vi "TBM.GetCallerCoordinates.vi"(8 "error in (no error)":errorcluster, 11 "Control in":refnum<vi>) -> (0 "error out":errorcluster, 1 "FP Screen Bounds":T1, 2 "Pane Color":u32, 3 "Ctrl Screen Bounds":T1)   [LabVIEW 2013, in "ToolbarMenu.lvlib"]
uses:
  ToolbarMenu.lvlib
  <vilib>/Utility/miscctls.llb/LVRectTypeDef.ctl
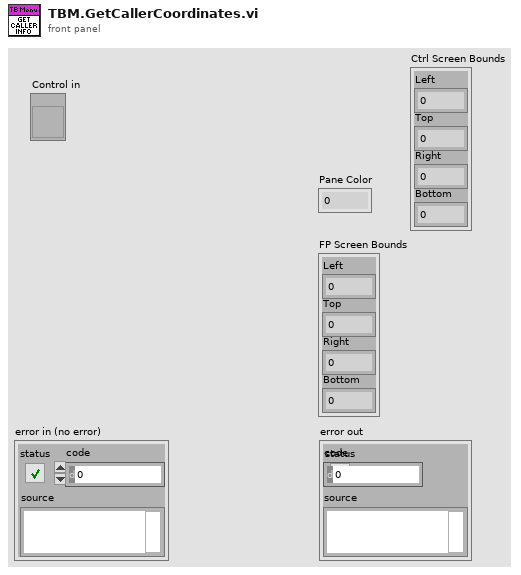
[diagram p1: front panel]
types:
  T1 = typedef "LVRectTypeDef.ctl" = cluster{"Left":i16, "Top":i16, "Right":i16, "Bottom":i16}
  T2 = typedef "LVPositionTypeDef.ctl" = cluster{"Left":i32, "Top":i32}
  T3 = typedef "LVBoundsTypeDef.ctl" = cluster{"Width":u32, "Height":u32}
  T4 = typedef "LVPointTypeDef.ctl" = cluster{"Horizontal":i16, "Vertical":i16}
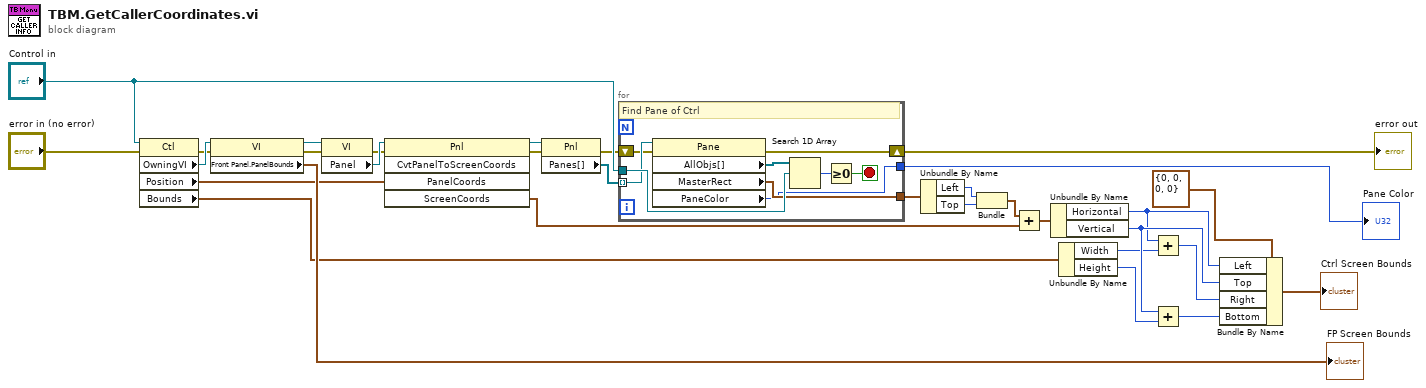
[diagram p0: block diagram]
diagram:
  n1 = property class="Ctl"(reference="Control in", error in="error in (no error)") -> (error out=w25:errorcluster, "OwningVI"=w27:refnum<vi>, "Position"=w21:T2, "Bounds"=w14:T3)  [unwired: 1 out]
  n2 = property class="VI"(reference=w27, error in=w25) -> (reference out=w26:refnum<vi>, error out=w24:errorcluster, "Front Panel.PanelBounds"=→"FP Screen Bounds":T1)
  n3 = property class="VI"(reference=w26, error in=w24) -> (error out=w3:errorcluster, "Panel"=w22:refnum<vi>)  [unwired: 1 out]
  n4 = invoke class="Pnl" method="CvtPanelToScreenCoords"(reference=w22, error in=w3, "PanelCoords"=w21) -> (reference out=w1:refnum<vi>, error out=w2:errorcluster, "ScreenCoords"=w9:T4)  [unwired: 2 in, 2 out]
  n5 = property on="Property Node" class="Pnl"(reference=w1, error in=w2) -> (error out=w29:errorcluster, "Panes[]"=w28:refnum<vi>[])  [unwired: 1 out]
  n6 = for {
    tunnel: w28 -> [w37] mode=indexing
    tunnel: "Control in" -> [w40]
    shift-right: [w34] -> w5
    shift-left: w29 -> [w33]
    tunnel: [w35] -> w12
    tunnel: [w32] -> w4
    stop <- w38 stop-if-true
    # "Find Pane of Ctrl"
    n7 = property class="Pane"(reference=w37, error in=w33) -> (error out=w34:errorcluster, "AllObjs[]"=w36:refnum<vi>[], "MasterRect"=w35:T1, "PaneColor"=w32:u32)  [unwired: 1 out]
    n8 = Search 1D Array(1D array=w36, element=w40) -> (index of element=w39:i32)  [unwired: 1 in]
    n9 = Greater Or Equal To 0?(x=w39) -> (x >= 0?=w38:bool)
  }
  "error out" <- w5
  "Pane Color" <- w4
  n10 = Unbundle By Name(w12) -> ("Left"=w11:i16, "Top"=w10:i16)
  n11 = Bundle("Left"=w11, "Top"=w10) -> (w7:cluster{"Left":i16, "Top":i16})  [unwired: 1 in]
  n12 = Add(x=w7, y=w9) -> (x+y=w8:T4)
  n13 = Unbundle By Name(w8) -> ("Horizontal"=w19:i16, "Vertical"=w20:i16)
  n14 = Unbundle By Name(w14) -> ("Width"=w16:u32, "Height"=w15:u32)
  n15 = Add(x=w19, y=w16) -> (x+y=w18:u32)
  n16 = Add(x=w20, y=w15) -> (x+y=w17:u32)
  n17 = Bundle By Name(cluster=T1 {"Left"=0, "Top"=0, "Right"=0, "Bottom"=0} ("Front Panel Window:Panel Bounds 2"), "Left"=w19, "Top"=w20, "Right"=w18, "Bottom"=w17) -> (→"Ctrl Screen Bounds":T1)
